vi "PID_calcule.vi"(6 "controlON":bool, 8 "Temperatura bobina":dbl format="%.2f", 9 "Temperatura manifold":dbl format="%.2f", 10 "Setpoint T":dbl, 11 "PID_Bitron.lvclass":refnum<class "PID_Bitron.lvclass">) -> (0 "PID_Bitron.lvclass out":refnum<class "PID_Bitron.lvclass">, 3 "PWM (%)":dbl)   [LabVIEW 2022 SP3, in "PID_Bitron.lvclass"]
uses:
  PID_Bitron.lvclass
  PID_Bitron.lvclass/PID_Bitron.ctl
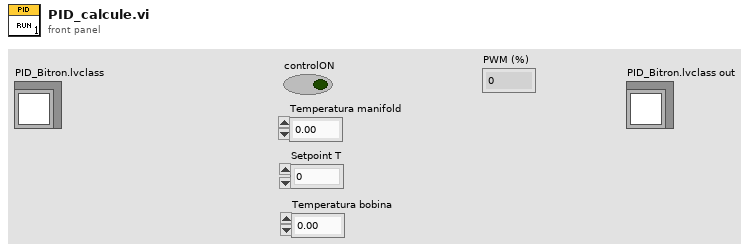
[diagram p1: front panel]
types:
  T1 = cluster{"proportional gain (Kc)":dbl, "integral time (Ti, min)":dbl, "derivative time (Td, min)":dbl}
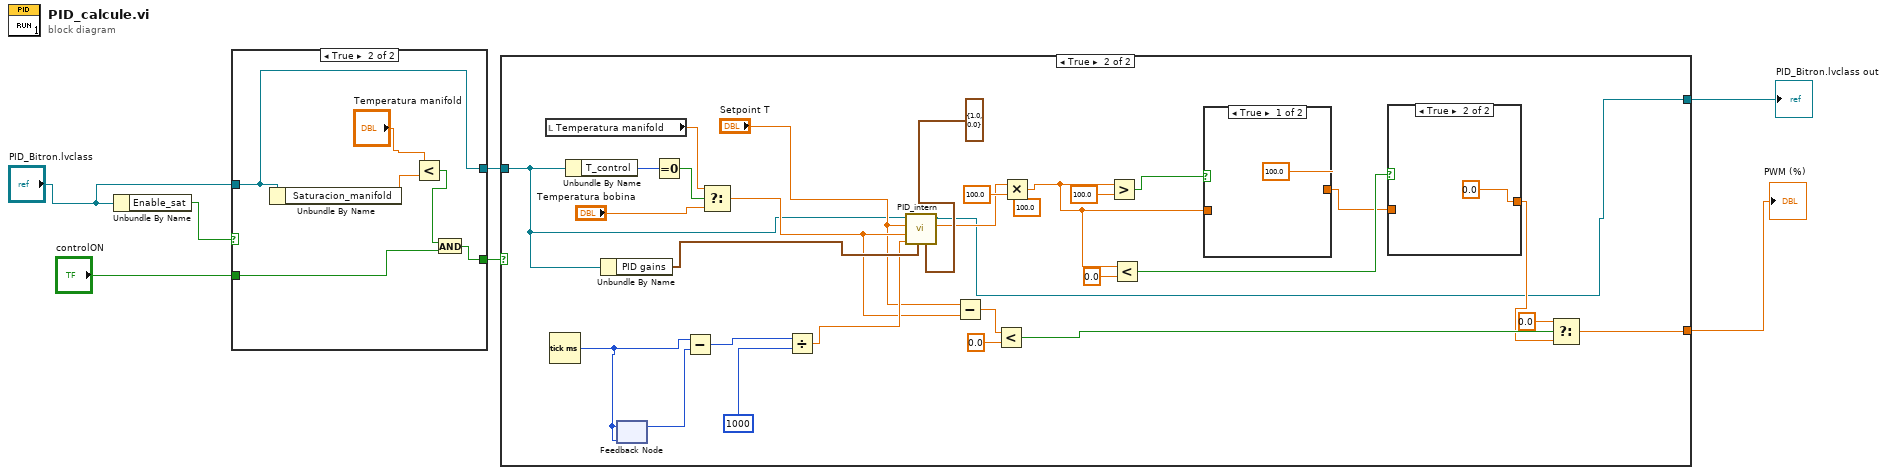
[diagram p0: block diagram]
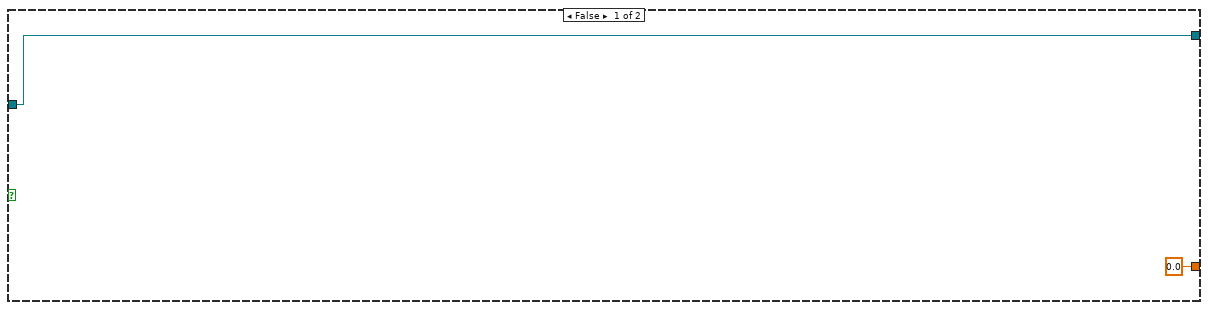
[diagram p3: hidden frame]
diagram:
  n1 = Unbundle By Name("PID_Bitron.lvclass") -> ("Enable_sat"=w4:bool)
  n2 = case shown="True" w4 {
    tunnel: [w9 w15] -> w7
    tunnel: "controlON" -> [w9 w14]
    tunnel: "PID_Bitron.lvclass" -> [w8 w10]
    tunnel: [w8 w10] -> w2
    frame False {
    }
    frame True {
      n3 = Unbundle By Name(w10) -> ("Saturacion_manifold"=w11:dbl)
      n4 = Less?(x="Temperatura manifold", y=w11) -> (x < y?=w12:bool)
      n5 = And(x=w12, y=w14) -> (x .and. y?=w15:bool)
    }
  }
  n6 = case shown="True" w7 {
    tunnel: [0.0 ("t") w30] -> w5
    tunnel: w2 -> [w16 w20]
    tunnel: [w16 w18] -> w1
    frame False {
    }
    frame True {
      (unwired) 100.0 ("y")
      n7 = local read "Temperatura manifold"() -> (w26:dbl)
      n8 = Tick Count (ms)() -> (millisecond timer value=w46:u32)
      n9 = Unbundle By Name(w20) -> ("T_control"=w28:enum16{"Manifold", "Bobina"})
      n10 = Unbundle By Name(w20) -> ("PID gains"=w24:T1)
      n11 = feedback #1(w46) -> (w45:u32)
      n12 = feedback-in #1(w46) -> ()
      n13 = Equal To 0?(x=w28) -> (x = 0?=w27:bool)
      n14 = Subtract(x=w46, y=w45) -> (x-y=w43:u32)
      n15 = Select(t=w26, s=w27, f="Temperatura bobina") -> (s? t:f=w22:dbl)
      n16 = Divide(x=w43, y=1000) -> (x/y=w23:dbl)
      n17 = call "PID_intern.vi"("output range"=cluster{"output high":dbl, "output low":dbl} {"output high"=1.0, "output low"=0.0}, "PID gains"=w24, "dt (s)"=w23, "process variable"=w22, "setpoint"="Setpoint T", "PID_Bitron.lvclass"=w20) -> ("output"=w19:dbl, "PID_Bitron.lvclass 2"=w18:refnum<class "PID_Bitron.lvclass">)  [unwired: 4 in]
      n18 = Subtract(x="Setpoint T", y=w22) -> (x-y=w35:dbl)
      n19 = Less?(x=w35, y=0.0) -> (x < y?=w33:bool)
      n20 = Multiply(x=w19, y=100.0) -> (x*y=w38:dbl)
      n21 = Greater?(x=w38, y=100.0) -> (0:w39:bool)
      n22 = Less?(x=w38, y=0.0) -> (x < y?=w37:bool)
      n23 = case shown="True" w39 {
        tunnel: w38 -> [_ w50]
        tunnel: [100.0 w50] -> w36
        frame True {
        }
        frame False {
        }
      }
      n24 = case shown="True" w37 {
        tunnel: w36 -> [w47 _]
        tunnel: [w47 0.0] -> w31
        frame False {
        }
        frame True {
        }
      }
      n25 = Select(t=0.0, s=w33, f=w31) -> (s? t:f=w30:dbl)
    }
  }
  "PWM (%)" <- w5
  "PID_Bitron.lvclass out" <- w1
